vi "Cannon Global.vi"() -> ()   [LabVIEW 2013]
uses:
  <vilib>/Rock Robotics/WPI/Solenoid/WPI_SolenoidValue.ctl
panel:
  in  "Cannon Info":T2
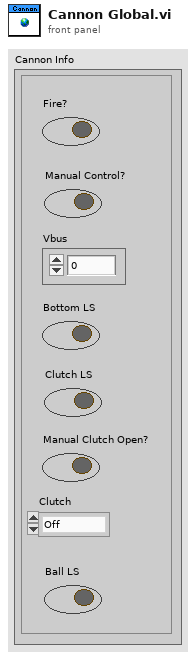
[diagram p1: front panel]
types:
  T1 = typedef "WPI_SolenoidValue.ctl" = enum16{"Off", "On", "Forward", "Reverse"}
  T2 = cluster{"Fire?":bool, "Manual Control?":bool, "Vbus":dbl, "Bottom LS":bool, "Clutch LS ":bool, "Manual Clutch Open?":bool, "Clutch":T1, "Ball LS":bool}
diagram:
